vi "Flatten Value.vi"(8 "error in (no error)":errorcluster, 11 "Boolean in":refnum<class "Boolean 1D.lvclass">) -> (0 "error out":errorcluster, 2 "Value":string, 3 "Boolean out":refnum<class "Boolean 1D.lvclass">)   [LabVIEW 2017, in "Boolean 1D.lvclass"]
uses:
  <vilib>/gpm_packages/@cs/data-type-serializer/source/Boolean 1D/Boolean 1D.lvclass
  <vilib>/gpm_packages/@cs/data-type-serializer/source/Boolean 1D/Boolean 1D.lvclass/Boolean 1D.ctl
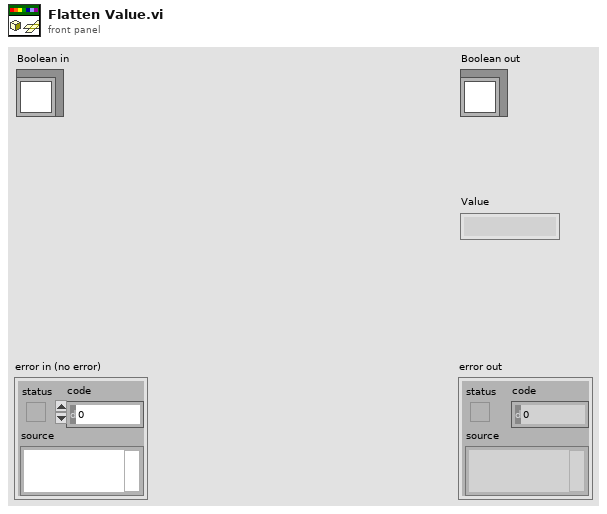
[diagram p1: front panel]
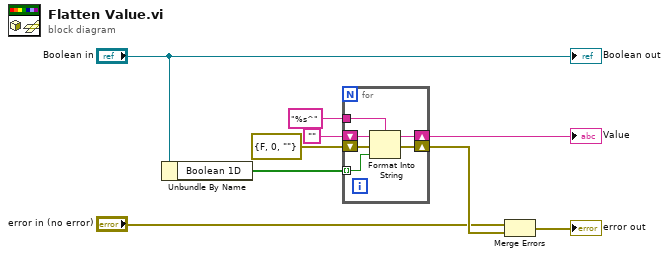
[diagram p0: block diagram]
diagram:
  n1 = Unbundle By Name("Boolean in") -> ("Boolean 1D"=w8:bool[])
  n2 = for {
    tunnel: w8 -> [w15] mode=indexing
    shift-right: [w14] -> w7
    shift-left: "" -> [w12]
    tunnel: "%s^" ("delimiter (Tab)") -> [w11]
    shift-right: [w13] -> w6
    shift-left: errorcluster {"status"=FALSE, "code"=0, "source"=""} ("error IO") -> [w10]
    n3 = Format Into String(format string=w11, initial string=w12, error in=w10, w15) -> (resulting string=w14:string, error out=w13:errorcluster)
  }
  "Value" <- w7
  n4 = Merge Errors("error in (no error)", w6) -> (→"error out":errorcluster)
  "Boolean out" <- "Boolean in"
